vi "Ler_pressao.vi"(4 "order":i32=2, 5 "low cutoff freq: fl":dbl=0.12500000000000006 format="%0.4f", 6 "high cutoff freq: fh":dbl=0.45000000000000007 format="%0.2f", 7 "filter type":T1, 10 "Statistic":T3(ring), 11 "intervals":i32=20) -> (0 "String":string, 1 "Data Set 2 Output":dbl format="%.3g", 2 "Data Set 1 Output":dbl format="%.3g", 3 "mean value pressao":dbl)   [LabVIEW 2011]
uses:
  <vilib>/Analysis/3filter.llb/Filter Passband Type.ctl
  <vilib>/DAQmx/read.llb/DAQmx Read (Analog 1D DBL 1Chan NSamp).vi
  <vilib>/DAQmx/create/channels.llb/DAQmx Create Channel (AI-Voltage-Basic).vi
  <vilib>/DAQmx/configure/timing.llb/DAQmx Timing (Sample Clock).vi
  <vilib>/DAQmx/miscellaneous.llb/DAQmx Fill In Error Info.vi
  <vilib>/Analysis/3filter.llb/Butterworth Filter (DBL).vi
  <vilib>/Analysis/baseanly.llb/Unimode.vi
  <vilib>/Analysis/5stat.llb/RMS (DBL).vi
  Program Files/National Instruments/LabVIEW 2011/resource/objmgr/daqmx.rc
  <vilib>/gmath/NI_Gmath.lvlib
  <vilib>/Analysis/NI_AALBase.lvlib
  <vilib>/Analysis/NI_AALPro.lvlib
panel:
  out "error":dbl
  out "?":T2(graph)
  out "Data Set 1":dbl[](graph)
  out "?":T2(graph)
  out "Data Set 2":dbl[](graph)
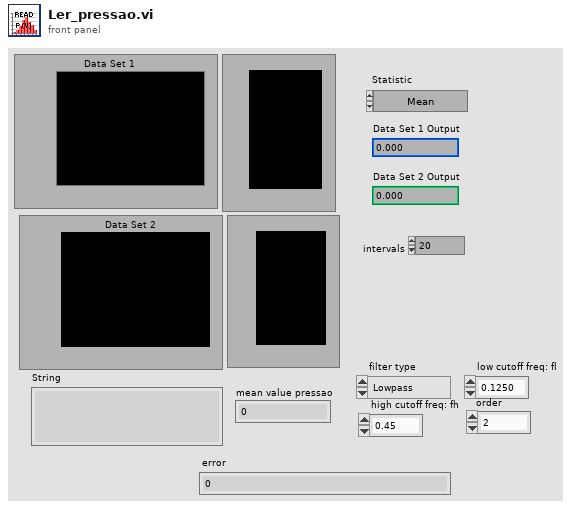
[diagram p1: front panel]
types:
  T1 = typedef "NI_AALBase.lvlib/Filter Passband Type.ctl" = enum32{"Lowpass", "Highpass", "Bandpass", "Bandstop"}
  T2 = cluster{"Histogram: h(x)":i32[], "X Values":dbl[]}
  T3 = enum16{"Mean", "Standard Deviation", "Variance", "Skewness", "Kurtosis", "Median", "Mode", "RMS"}
  T4 = enum16{"arithmetic", "geometric", "harmonic", "trimmed", "median"}
  T5 = cluster{"intervals":i32, "Statistic":enum16{"Mean", "Standard Deviation", "Variance", "Skewness", "Kurtosis", "Median", "Mode", "RMS"}}
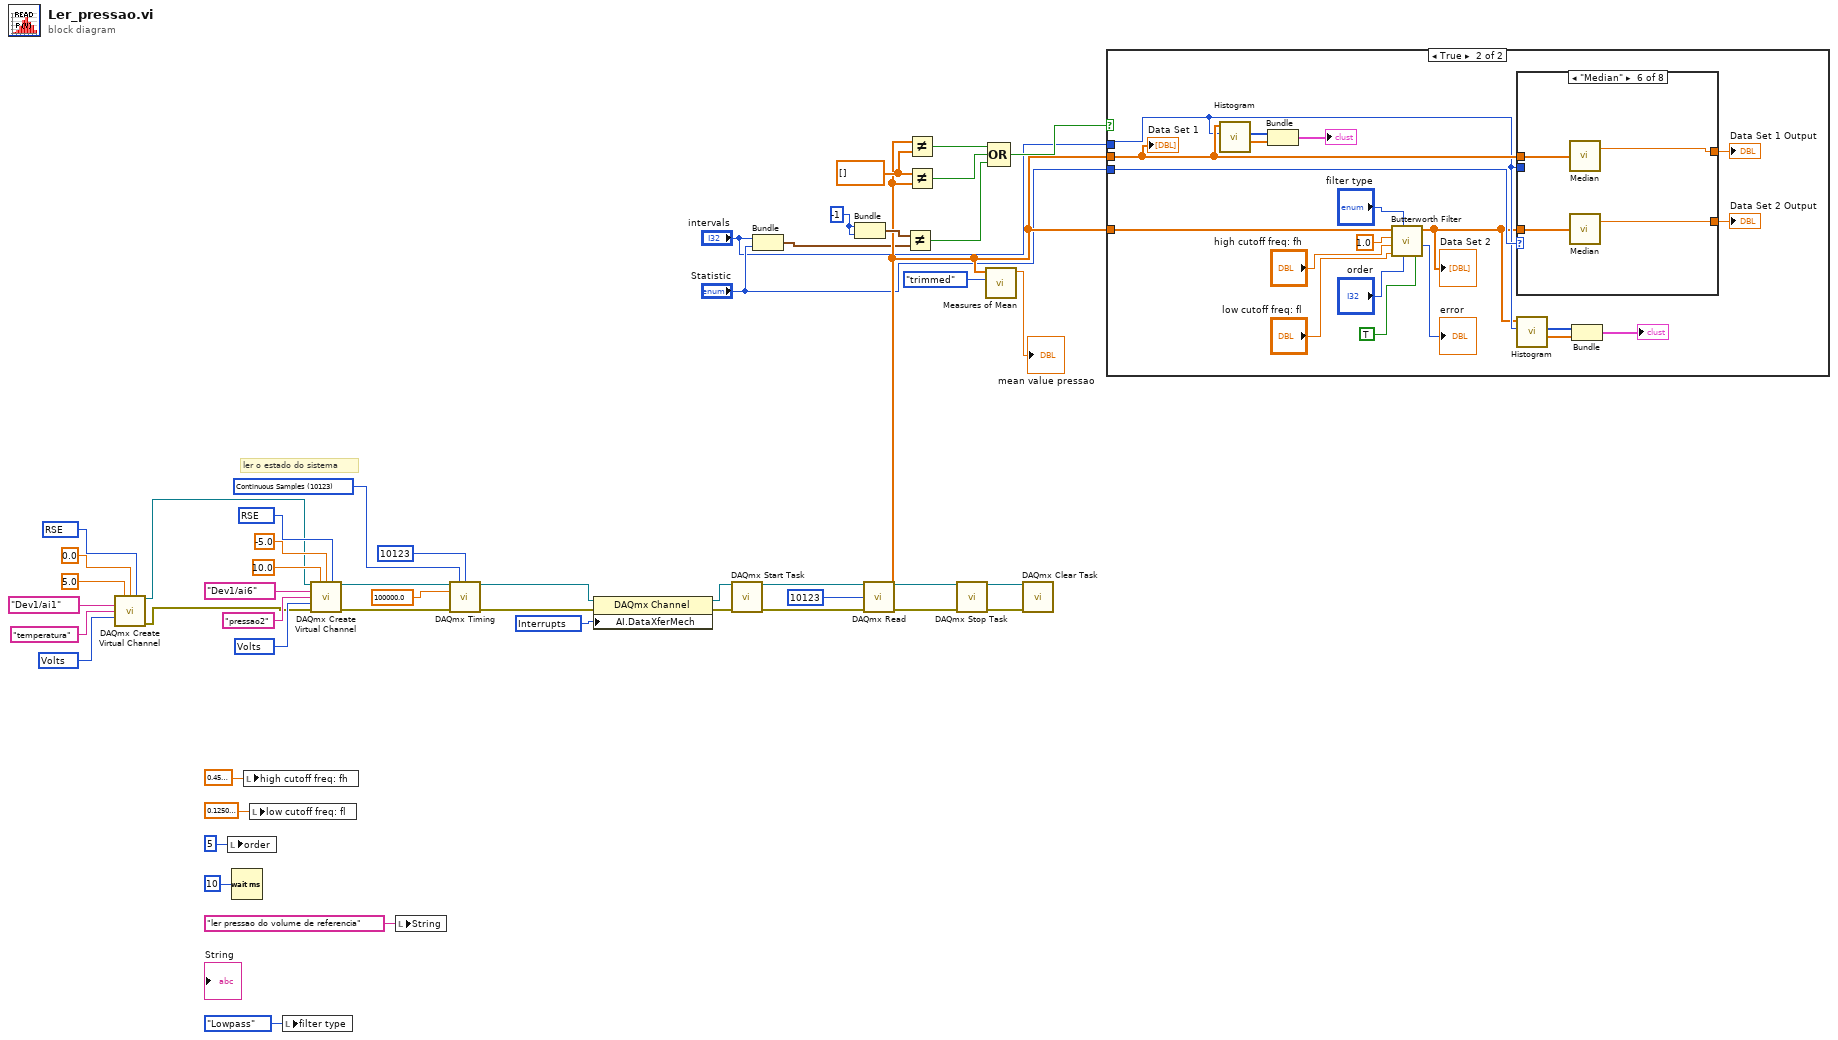
[diagram p0: block diagram]
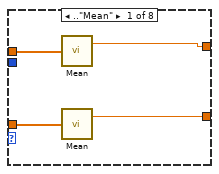
[diagram p3: hidden frame]
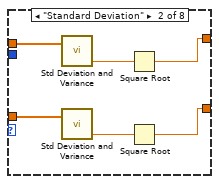
[diagram p4: hidden frame]
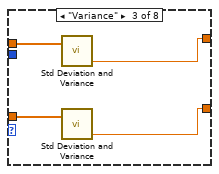
[diagram p5: hidden frame]
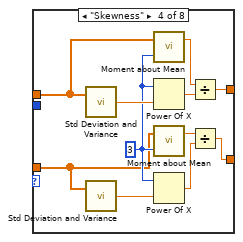
[diagram p6: hidden frame]
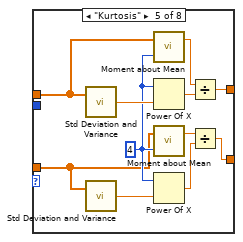
[diagram p7: hidden frame]
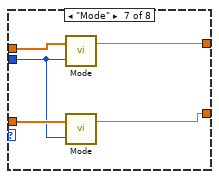
[diagram p8: hidden frame]
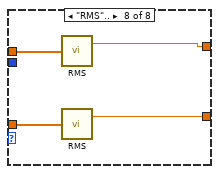
[diagram p9: hidden frame]
diagram:
  w6 = 10083 items=["default"=-1, "RSE"=10083, "NRSE"=10078, "Differential"=10106, "Pseudodifferential"=12529] ("input terminal configuration")
  w7 = 10348 items=["Volts"=10348, "From Custom Scale"=10065] ("units")
  w24 = dbl[] []
  w22 = -1
  w41 = 10204 items=["DMA"=10054, "Interrupts"=10204, "Programmed I/O"=10264, "USB Bulk"=12590] ("AI.DataXferMech")
  w44 = 10123 items=["Finite Samples"=10178, "Continuous Samples"=10123, "Hardware Timed Single Point"=12522] ("sample mode")
  w48 = 10083 items=["default"=-1, "RSE"=10083, "NRSE"=10078, "Differential"=10106, "Pseudodifferential"=12529] ("input terminal configuration")
  w49 = 10348 items=["Volts"=10348, "From Custom Scale"=10065] ("units")
  # "ler o estado do sistema"
  n1 = call-poly <vilib>:"DAQmx Create Virtual Channel.vi"("maximum value"=5.0, "minimum value"=0.0, "input terminal configuration"=w6, "physical channels"=tag "Dev1/ai1" ("P S1"), "name to assign"="temperatura", "units"=w7) -> ("task out"=w2:refnum<k21>, "error out"=w1:errorcluster)  [unwired: 8 in]
  n2 = local write "order"(5 ("order")) -> ()
  n3 = Wait (ms)(milliseconds to wait=u32 10) -> ()  [unwired: 1 out]
  n4 = local write "high cutoff freq: fh"(0.45000000000000007 ("high cutoff freq: fh")) -> ()
  n5 = local write "low cutoff freq: fl"(0.12500000000000006 ("low cutoff freq: fl")) -> ()
  n6 = local write "filter type"(Filter_Passband_Type."Lowpass" ("filter type")) -> ()
  n7 = call-poly <vilib>:"DAQmx Create Virtual Channel.vi"("task in"=w2, "maximum value"=10.0, "minimum value"=-5.0, "input terminal configuration"=w48, "physical channels"=tag "Dev1/ai6" ("P S1"), "name to assign"="pressao2", "units"=w49, "error in"=w1) -> ("task out"=w38:refnum<k21>, "error out"=w37:errorcluster)  [unwired: 6 in]
  n8 = local write "String"("ler pressao do volume de referencia" ("String")) -> ()
  n9 = call-poly <vilib>:"DAQmx Timing.vi"("task/channels in"=w38, "sample mode"=w44, "samples per channel"=10123, "rate"=100000.0, "error in"=w37) -> ("task out"=w43:refnum<k21>, "error out"=w42:errorcluster)  [unwired: 9 in]
  n10 = property class="DAQmx Channel"(reference=w43, error in=w42, "AI.DataXferMech"=w41) -> (reference out=w40:refnum<k21>, error out=w39:errorcluster)
  n11 = call <vilib>:"DAQmx Start Task.vi"("task/channels in"=w40, "error in"=w39) -> ("task out"=w46:refnum<k21>, "error out"=w45:errorcluster)  [unwired: 12 in]
  n12 = Bundle("intervals"="intervals", "Statistic"="Statistic") -> (w16:T5)  [unwired: 1 in]
  n13 = Bundle(w22, w22) -> (w23:cluster{i32, i32})  [unwired: 1 in]
  n14 = call-poly <vilib>:"DAQmx Read.vi"("task/channels in"=w46, "number of samples per channel"=10123, "error in"=w45) -> ("task out"=w30:refnum<k21>, "data"=w21:dbl[], "error out"=w28:errorcluster)  [unwired: 10 in]
  n15 = Not Equal?(x=w23, y=w16) -> (x != y?=w15:bool)
  n16 = Not Equal?(x=w21, y=w24) -> (x != y?=w19:bool)
  n17 = Not Equal?(x=w24, y=w21) -> (x != y?=w18:bool)
  n18 = call <vilib>:"DAQmx Stop Task.vi"("task/channels in"=w30, "error in"=w28) -> ("task out"=w29:refnum<k21>, "error out"=w27:errorcluster)  [unwired: 12 in]
  n19 = call <vilib>:"Measures of Mean.vi"("type"=T4."trimmed", "x array"=w21) -> ("mean value"=→"mean value pressao":dbl)  [unwired: 8 in, 1 out]
  n20 = Compound Arithmetic op=OR(w19, w18, w15) -> (w20:bool)
  n21 = call <vilib>:"DAQmx Clear Task.vi"("task in"=w29, "error in"=w27) -> ()  [unwired: 13 in, 1 out]
  n22 = case shown="True" w20 {
    tunnel: w21 -> [_ w57]
    tunnel: w21 -> [_ w66]
    tunnel: "Statistic" -> [_ w68]
    tunnel: "intervals" -> [_ w64]
    frame False {
    }
    frame True {
      n23 = call <vilib>:"Histogram.vi"("intervals"=w64, "X"=w66) -> ("X Values"=w62:dbl[], "Histogram: h(x)"=w63:i32[])  [unwired: 6 in, 2 out]
      n24 = Bundle("Histogram: h(x)"=w63, "X Values"=w62) -> (→"?":T2)  [unwired: 1 in]
      n25 = call-poly <vilib>:"Butterworth Filter.vi"("init/cont (init:F)"=TRUE, "order"="order", "filter type"="filter type", "low cutoff freq: fl"="low cutoff freq: fl", "high cutoff freq: fh"="high cutoff freq: fh", "sampling freq: fs"=1.0, "X"=w57) -> ("error"=→"error":i32, "Filtered X"=w56:dbl[])  [unwired: 1 in]
      "Data Set 2" <- w56
      n26 = case shown="\"Median\"" w68 {
        tunnel: w56 -> [w74 w79 w83 w90 w101 w110 w115 w119]
        tunnel: [w72 w76 w82 w87 w98 w108 w113 w118] -> w69
        tunnel: [w73 w80 w84 w91 w102 w109 w114 w117] -> w70
        tunnel: w66 -> [w71 w75 w81 w94 w105 w107 w112 w116]
        tunnel: w64 -> [_ _ _ _ _ _ w111 _]
        frame .."Mean" {
          n27 = call <vilib>:"Mean.vi"("X"=w71) -> ("mean"=w73:dbl)  [unwired: 1 out]
          n28 = call <vilib>:"Mean.vi"("X"=w74) -> ("mean"=w72:dbl)  [unwired: 1 out]
        }
        frame "Standard Deviation" {
          n29 = call <vilib>:"Std Deviation and Variance.vi"("X"=w75) -> ("variance"=w78:dbl)  [unwired: 1 in, 2 out]
          n30 = call <vilib>:"Std Deviation and Variance.vi"("X"=w79) -> ("variance"=w77:dbl)  [unwired: 1 in, 2 out]
          n31 = Square Root(x=w78) -> (sqrt(x)=w80:dbl)
          n32 = Square Root(x=w77) -> (sqrt(x)=w76:dbl)
        }
        frame "Variance" {
          n33 = call <vilib>:"Std Deviation and Variance.vi"("X"=w81) -> ("variance"=w84:dbl)  [unwired: 1 in, 2 out]
          n34 = call <vilib>:"Std Deviation and Variance.vi"("X"=w83) -> ("variance"=w82:dbl)  [unwired: 1 in, 2 out]
        }
        frame "Skewness" {
          w92 = 3
          n35 = call <vilib>:"Std Deviation and Variance.vi"("X"=w94) -> ("standard deviation"=w95:dbl)  [unwired: 1 in, 2 out]
          n36 = call <vilib>:"Std Deviation and Variance.vi"("X"=w90) -> ("standard deviation"=w93:dbl)  [unwired: 1 in, 2 out]
          n37 = call <vilib>:"Moment about Mean.vi"("order"=w92, "X"=w94) -> ("moment"=w85:dbl)  [unwired: 1 out]
          n38 = Power Of X(1:w95, 2:w92) -> (0:w86:dbl)
          n39 = call <vilib>:"Moment about Mean.vi"("order"=w92, "X"=w90) -> ("moment"=w88:dbl)  [unwired: 1 out]
          n40 = Power Of X(1:w93, 2:w92) -> (0:w89:dbl)
          n41 = Divide(x=w85, y=w86) -> (x/y=w91:dbl)
          n42 = Divide(x=w88, y=w89) -> (x/y=w87:dbl)
        }
        frame "Kurtosis" {
          w103 = 4
          n43 = call <vilib>:"Std Deviation and Variance.vi"("X"=w105) -> ("standard deviation"=w106:dbl)  [unwired: 1 in, 2 out]
          n44 = call <vilib>:"Std Deviation and Variance.vi"("X"=w101) -> ("standard deviation"=w104:dbl)  [unwired: 1 in, 2 out]
          n45 = call <vilib>:"Moment about Mean.vi"("order"=w103, "X"=w105) -> ("moment"=w97:dbl)  [unwired: 1 out]
          n46 = Power Of X(1:w106, 2:w103) -> (0:w96:dbl)
          n47 = call <vilib>:"Moment about Mean.vi"("order"=w103, "X"=w101) -> ("moment"=w99:dbl)  [unwired: 1 out]
          n48 = Power Of X(1:w104, 2:w103) -> (0:w100:dbl)
          n49 = Divide(x=w97, y=w96) -> (x/y=w102:dbl)
          n50 = Divide(x=w99, y=w100) -> (x/y=w98:dbl)
        }
        frame "Median" {
          n51 = call <vilib>:"Median.vi"("X"=w107) -> ("median"=w109:dbl)  [unwired: 1 out]
          n52 = call <vilib>:"Median.vi"("X"=w110) -> ("median"=w108:dbl)  [unwired: 1 out]
        }
        frame "Mode" {
          n53 = call-poly <vilib>:"Mode.vi"("intervals"=w111, "X"=w112) -> ("mode"=w114:dbl)  [unwired: 1 out]
          n54 = call-poly <vilib>:"Mode.vi"("intervals"=w111, "X"=w115) -> ("mode"=w113:dbl)  [unwired: 1 out]
        }
        frame "RMS".. {
          n55 = call-poly <vilib>:"RMS.vi"("X"=w116) -> ("rms value"=w117:dbl)  [unwired: 1 out]
          n56 = call-poly <vilib>:"RMS.vi"("X"=w119) -> ("rms value"=w118:dbl)  [unwired: 1 out]
        }
      }
      "Data Set 1 Output" <- w70
      "Data Set 2 Output" <- w69
      n57 = call <vilib>:"Histogram.vi"("intervals"=w64, "X"=w56) -> ("X Values"=w60:dbl[], "Histogram: h(x)"=w61:i32[])  [unwired: 6 in, 2 out]
      n58 = Bundle("Histogram: h(x)"=w61, "X Values"=w60) -> (→"?":T2)  [unwired: 1 in]
      "Data Set 1" <- w66
    }
  }
